vi "iteration_graph_update.vi"(7 "Iteration Graph Settings":T1, 8 "error in (no error)":errorcluster, 9 "Iteration Number":i32, 10 "ROI Array In":dbl[][][](array[numeric]), 11 "GUI refnum cluster":T2) -> (0 "error out":errorcluster, 2 "Waveform Graph":dbl[][](graph))   [LabVIEW 2013]
uses:
  gui_refnum.ctl
  DDS drivers v3/Array_of_DDS_Boxes.ctl
  DDS drivers v3/DDS_box_cluster.ctl
  DDS drivers v3/DDS_box_device_reference.ctl
  <vilib>/ni845x/ni845x.llb/ni845xControl.ctl
  DDS drivers v3/array_of_DDS_channels.ctl
  DDS drivers v3/DDS_channel.ctl
  DDS drivers v3/array_of_DDS_profiles.ctl
  DDS drivers v3/DDS_profile.ctl
  DDS drivers v3/DDS RAM mode.ctl
  Counter/counter_graph_refnums.ctl
  gui_execution_controls.ctl
  PI_piezo/status.ctl
  PI_piezo/PI_Piezo.lvclass
  DDS/DDS.lvclass
panel:
  in  "Iteration Graph Array":dbl[][](array[numeric])
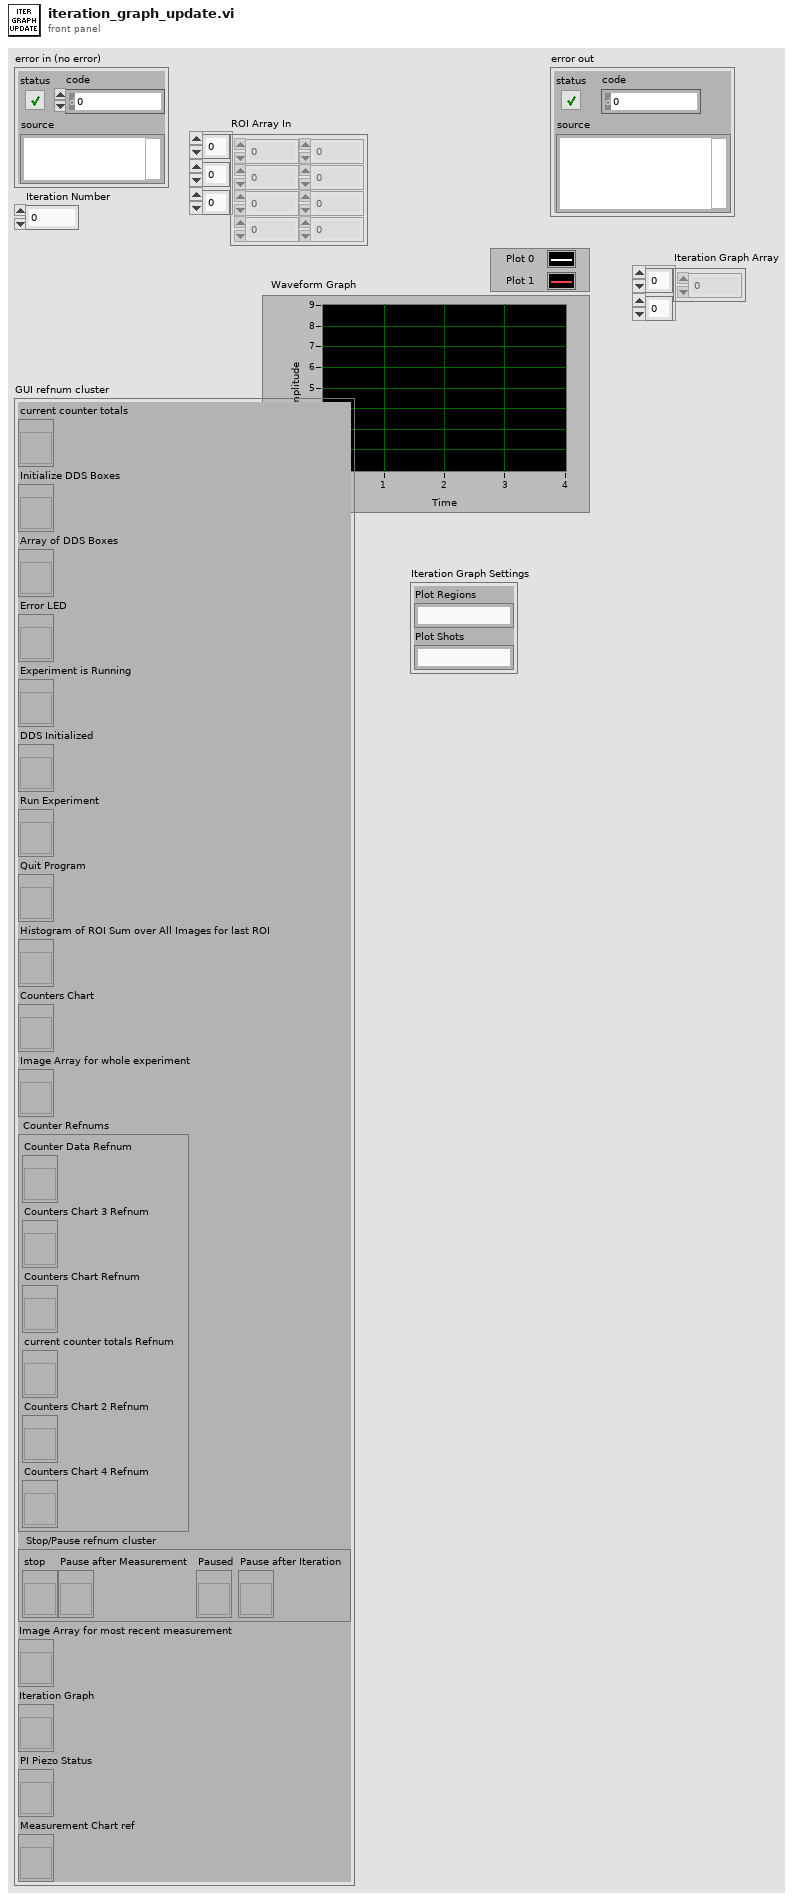
[diagram p1: front panel]
types:
  T1 = cluster{"Plot Regions":string, "Plot Shots":string}
  T2 = typedef "gui_refnum.ctl" = cluster{"current counter totals":refnum<vi>, "Initialize DDS Boxes":refnum<vi>, "Array of DDS Boxes":refnum<vi>, "Error LED":refnum<vi>, "Experiment is Running":refnum<vi>, "DDS Initialized":refnum<vi>, "Run Experiment":refnum<vi>, "Quit Program":refnum<vi>, "Histogram of ROI Sum over All Images for last ROI":refnum<vi>, "Counters Chart":refnum<vi>, "Image Array for whole experiment":refnum<vi>, "Counter Refnums":T3, "Stop/Pause refnum cluster":T4, "Image Array for most recent measurement":refnum<vi>, "Iteration Graph":refnum<vi>, "PI Piezo Status":refnum<vi>, "Measurement Chart ref":refnum<vi>}
  T3 = typedef "counter_graph_refnums.ctl" = cluster{"Counter Data Refnum":refnum<vi>, "Counters Chart 3 Refnum":refnum<vi>, "Counters Chart Refnum":refnum<vi>, "current counter totals Refnum":refnum<vi>, "Counters Chart 2 Refnum":refnum<vi>, "Counters Chart 4 Refnum":refnum<vi>}
  T4 = typedef "gui_execution_controls.ctl" = cluster{"stop":refnum<vi>, "Pause after Measurement":refnum<vi>, "Paused":refnum<vi>, "Pause after Iteration":refnum<vi>}
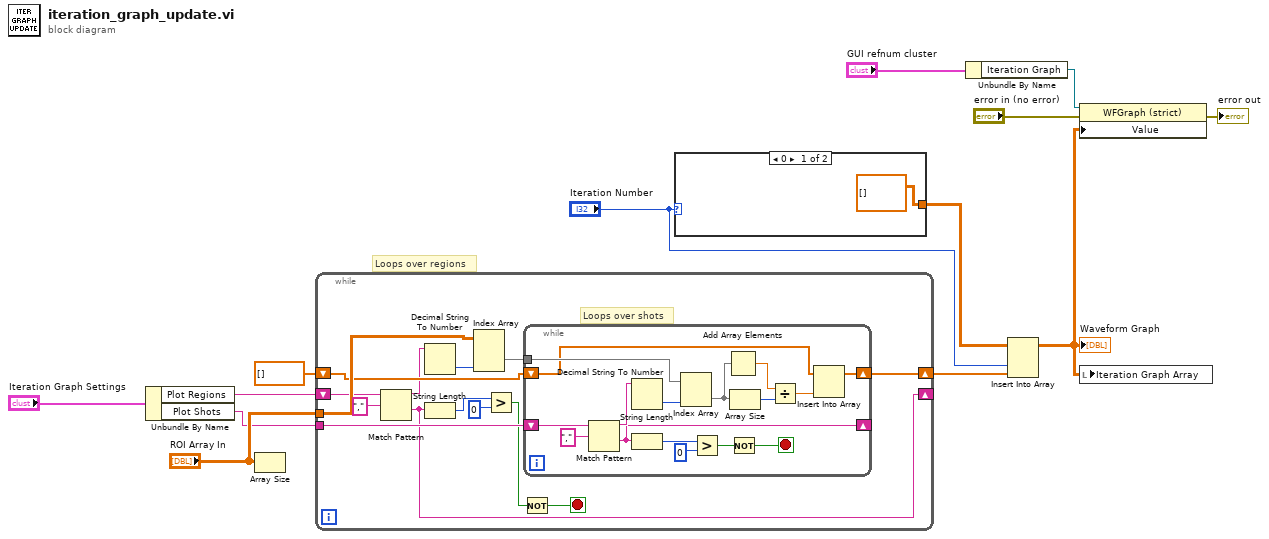
[diagram p0: block diagram]
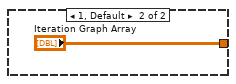
[diagram p2: hidden frame]
diagram:
  # "Loops over regions"
  n1 = Unbundle By Name("Iteration Graph Settings") -> ("Plot Regions"=w2:string, "Plot Shots"=w1:string)
  n2 = Array Size(array="ROI Array In") -> ()  [unwired: 1 out]
  n3 = while {
    tunnel: "ROI Array In" -> [w27]
    shift-right: [w26] -> w5
    shift-left: dbl[] [] ("array") -> [w24]
    shift-right: [w18] -> _
    shift-left: w2 -> [w23]
    tunnel: w1 -> [w20]
    stop <- w14 stop-if-true
    # "Loops over shots"
    n4 = Match Pattern(string=w23, regular expression=",") -> (before substring=w21:string, after substring=w18:string)  [unwired: 1 in, 2 out]
    n5 = Decimal String To Number(string=w21) -> (number=w19:i32)  [unwired: 2 in, 1 out]
    n6 = String Length(string=w18) -> (length=w17:i32)
    n7 = Index Array(array=w27, index (dim 2)=w19) -> (element=w25:dbl[][])  [unwired: 2 in]
    n8 = Greater?(x=w17, y=0) -> (0:w15:bool)
    n9 = Not(x=w15) -> (.not. x?=w14:bool)
    n10 = while {
      tunnel: w25 -> [w43]
      shift-right: [w42] -> w26
      shift-left: w24 -> [w41]
      shift-right: [w30] -> _
      shift-left: w20 -> [w39]
      stop <- w28 stop-if-true
      n11 = Match Pattern(string=w39, regular expression=",") -> (before substring=w40:string, after substring=w30:string)  [unwired: 1 in, 2 out]
      n12 = Decimal String To Number(string=w40) -> (number=w37:i32)  [unwired: 2 in, 1 out]
      n13 = String Length(string=w30) -> (length=w32:i32)
      n14 = Index Array(array=w43, index (col)=w37) -> (element=w35:dbl[])  [unwired: 1 in]
      n15 = Greater?(x=w32, y=0) -> (0:w29:bool)
      n16 = Add Array Elements(numeric array=w35) -> (sum=w34:dbl)
      n17 = Not(x=w29) -> (.not. x?=w28:bool)
      n18 = Array Size(array=w35) -> (size(s)=w36:i32)
      n19 = Divide(x=w34, y=w36) -> (x/y=w33:dbl)
      n20 = Insert Into Array(array=w41, new element=w33) -> (w42:dbl[])  [unwired: 1 in]
    }
  }
  n21 = case shown="0" "Iteration Number" {
    tunnel: [dbl[][] [] "Iteration Graph Array"] -> w8
    frame 0 {
    }
    frame 1, Default {
    }
  }
  n22 = Unbundle By Name("GUI refnum cluster") -> ("Iteration Graph"=w11:refnum<vi>)
  n23 = Insert Into Array(array=w8, index (col)="Iteration Number", new element=w5) -> (w4:dbl[][])  [unwired: 1 in]
  "Waveform Graph" <- w4
  n24 = property class="WFGraph (strict)"(reference=w11, error in="error in (no error)", "Value"=w4) -> (error out=→"error out":errorcluster)  [unwired: 1 out]
  n25 = local write "Iteration Graph Array"(w4) -> ()
